vi "quicktest_one_inst.vi"() -> ()   [LabVIEW 2009]
panel:
  out "bucle":i32
  out "Numeric":i32
  out "hex integer string 2":string
  out "IPR value 2":i32
  in  "send continuous":bool
  out "Data out 5":string
  in  "send":bool
  out "hex integer string":string
  out "IPR value":i32
  out "Id in":i32=72
  in  "Read physical":bool
  out "Data to send hex":string
  in  "Register or channel":i32=72
  in  "Device":u16(ring) items=["Attenuation", "Clipping", "Enable channel", "Delay line", "ASIC"]
  in  "Read/#write":bool
  out "data out serial":string
  out "Data to send dec":u32
  in  "Data":i32=72
  out "data out 2":string
  out "error out":errorcluster
  in  "stop":bool
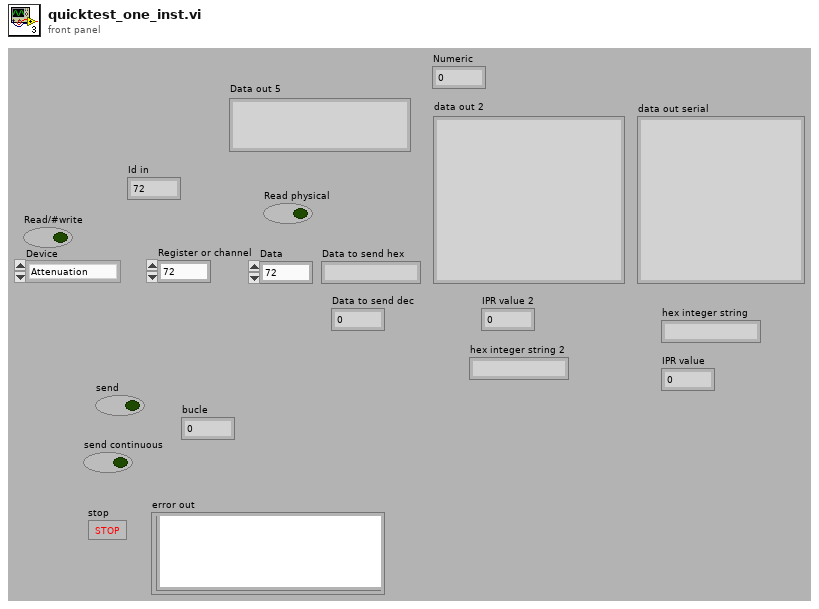
[diagram p1: front panel]
types:
  T1 = enum16{"Standard", "Buffered", "CRLF", "Immediate"}
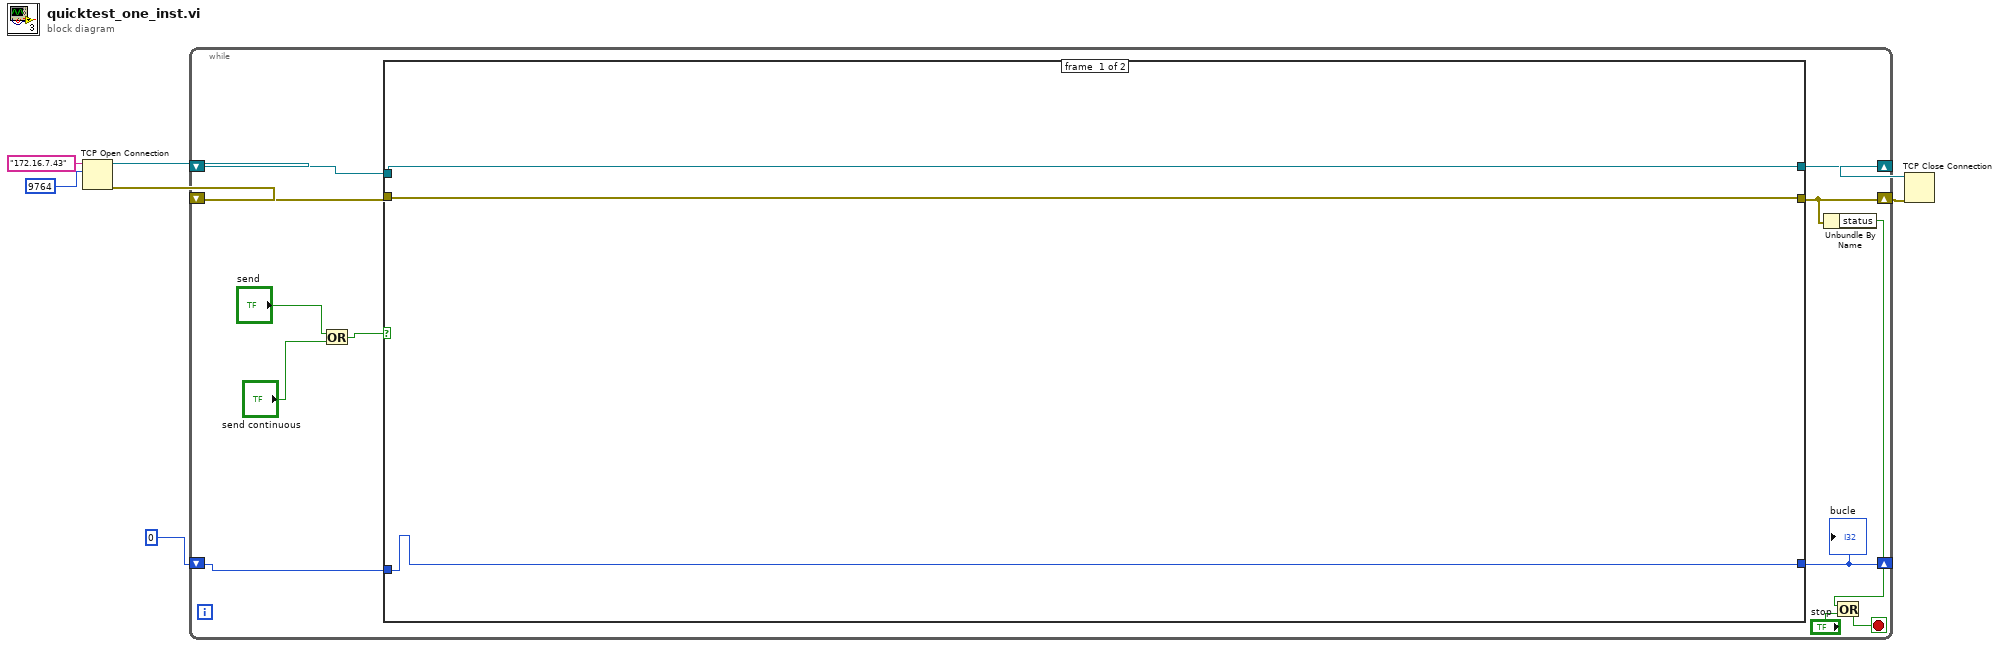
[diagram p0: block diagram]
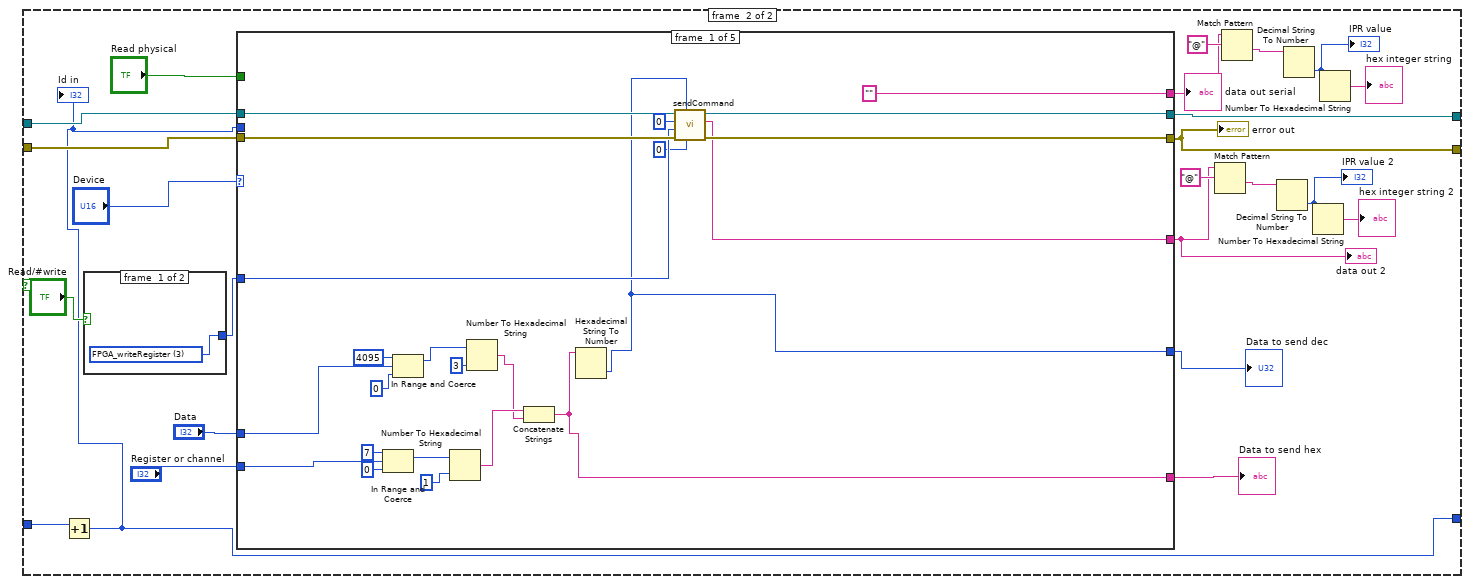
[diagram p2: hidden frame]
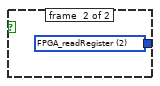
[diagram p3: hidden frame]
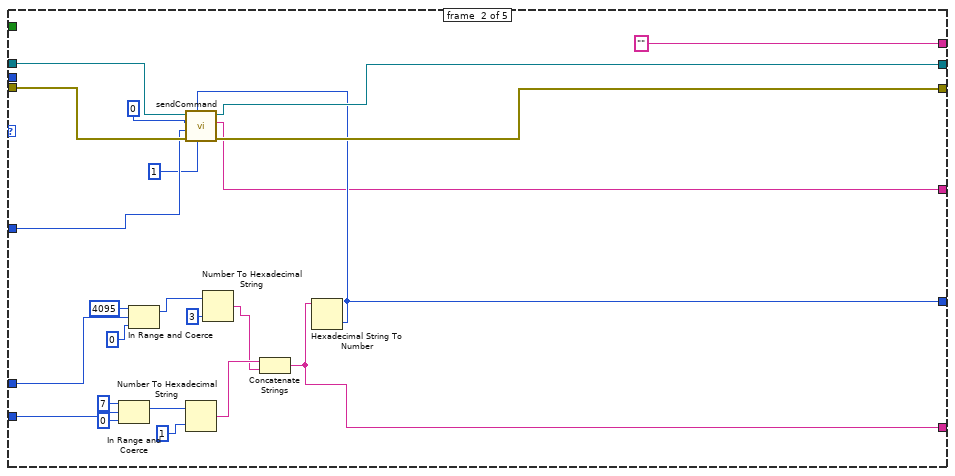
[diagram p4: hidden frame]
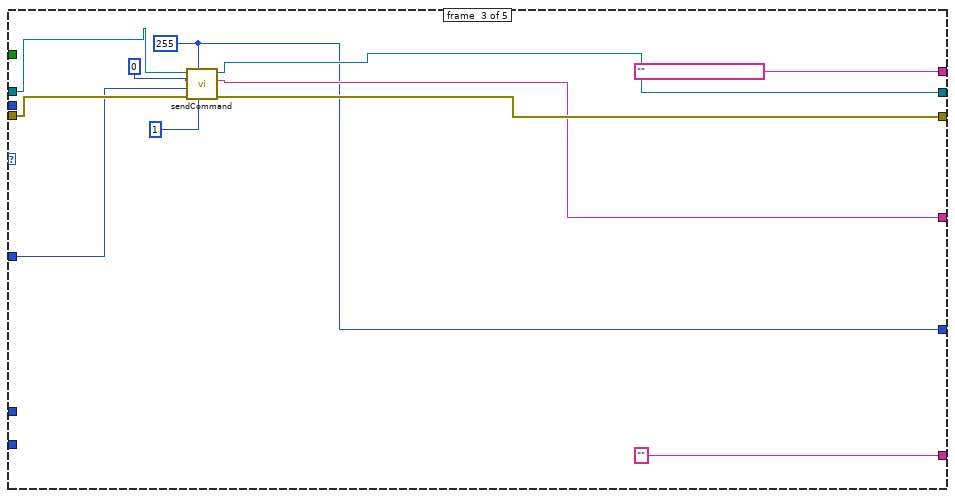
[diagram p5: hidden frame]
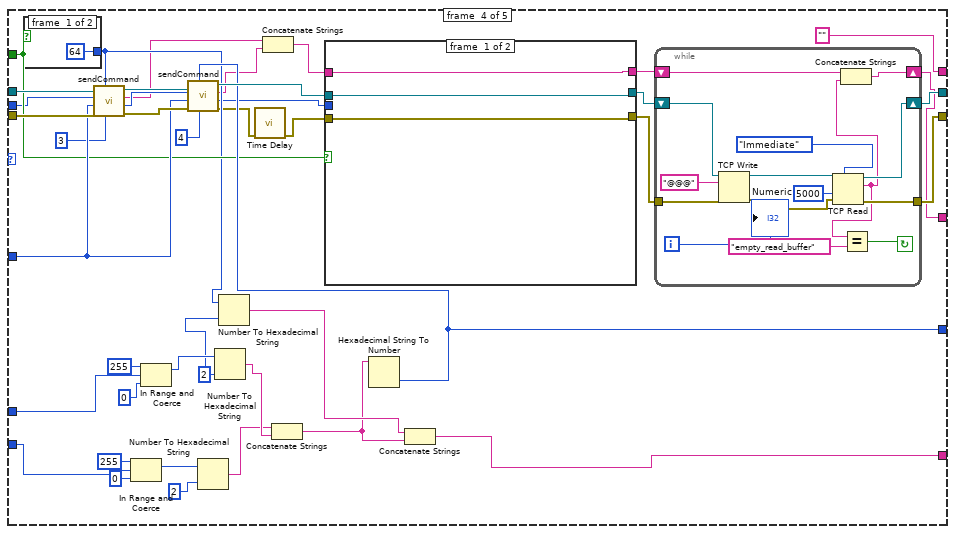
[diagram p6: hidden frame]
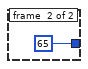
[diagram p7: hidden frame]
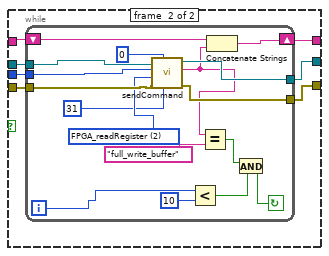
[diagram p8: hidden frame]
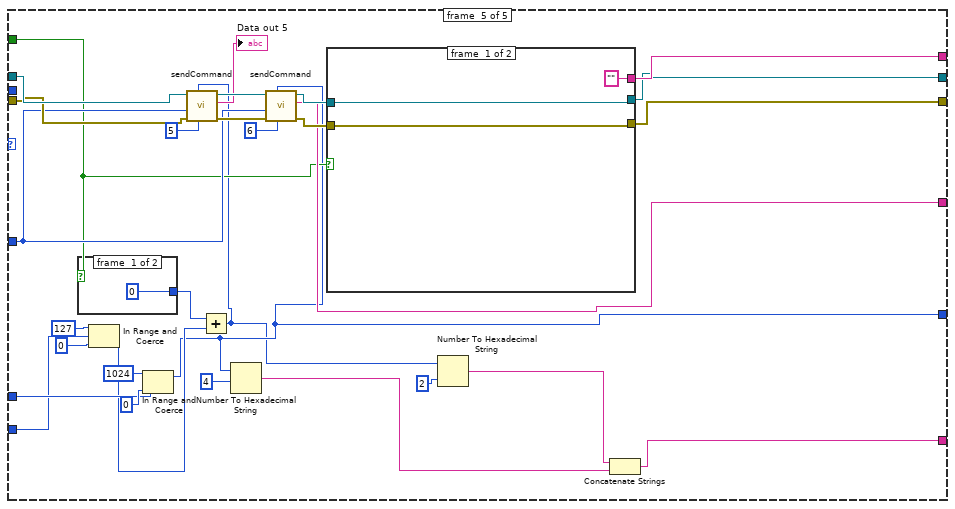
[diagram p9: hidden frame]
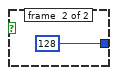
[diagram p10: hidden frame]
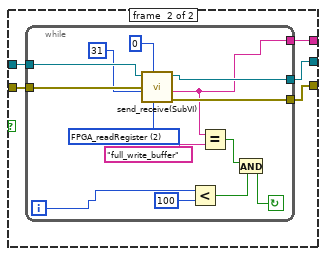
[diagram p11: hidden frame]
diagram:
  n1 = TCP Open Connection(address="172.16.7.43", remote port or service name=u16 9764) -> (connection ID=w3:refnum<k5>, error out=w2:errorcluster)  [unwired: 3 in]
  n2 = while {
    shift-right: [w18] -> w5
    shift-left: w2 -> [w13]
    shift-right: [w19] -> w4
    shift-left: w3 -> [w14]
    shift-right: [w9] -> _
    shift-left: 0 ("lower limit") -> [w8]
    stop <- w17 stop-if-true
    n3 = Or(x="send", y="send continuous") -> (x .or. y?=w10:bool)
    n4 = case shown="True" w10 {
      tunnel: w13 -> [w21 w46]
      tunnel: w14 -> [w22 w45]
      tunnel: [w22 w44] -> w19
      tunnel: [w21 w43] -> w18
      tunnel: [w20 w23] -> w9
      tunnel: w8 -> [w20 w24]
      frame #0 {
      }
      frame #1 {
        n5 = Increment(x=w24) -> (x+1=w23:i32)
        "Id in" <- w23
        n6 = case shown="False" "Read/#write" {
          tunnel: [w47 w48] -> w41
          frame #0 {
            w47 = u16 3 items=["sendCommand"=9, "FPGA_writeRegister"=3, "FPGA_readRegister"=2, "uC_writeRegister"=1, "uC_readRegister"=0] ("Action")
          }
          frame #1 {
            w48 = u16 2 items=["sendCommand"=9, "FPGA_writeRegister"=3, "FPGA_readRegister"=2, "uC_writeRegister"=1, "uC_readRegister"=0] ("Action")
          }
        }
        n7 = case shown="3" "Device" {
          tunnel: [w69 w92 w100 w113 w198] -> w43
          tunnel: w46 -> [w70 w94 w103 w146 w205]
          tunnel: w45 -> [w71 w93 w102 w143 w206]
          tunnel: [w68 w91 w101 w114 w199] -> w44
          tunnel: w41 -> [w56 w88 w97 w142 w204]
          tunnel: "Register or channel" -> [w49 w87 _ w130 w202]
          tunnel: "Data" -> [w50 w82 _ w129 w203]
          tunnel: ["" ("data out") "" ("data out") "" ("data out") "" ("data out") w200] -> w32
          tunnel: [w53 w75 w96 w128 w192] -> w37
          tunnel: [w52 w74 "" w118 w201] -> w36
          tunnel: [w54 w73 w99 w108 w197] -> w25
          tunnel: "Read physical" -> [_ _ _ w127 w196]
          tunnel: w23 -> [_ _ _ w117 _]
          frame #0 {
            n8 = In Range and Coerce(upper limit=7, x=w49, lower limit=0) -> (coerced(x)=w66:i32)  [unwired: 1 out]
            n9 = In Range and Coerce(upper limit=4095, x=w50, lower limit=0) -> (coerced(x)=w62:i32)  [unwired: 1 out]
            n10 = Number To Hexadecimal String(1:i16 1 ("width (-)"), 2:w66) -> (0:w59:string)
            n11 = Number To Hexadecimal String(1:i16 3 ("width (-)"), 2:w62) -> (0:w58:string)
            n12 = Concatenate Strings(w59, w58) -> (w52:string)
            n13 = Hexadecimal String To Number(string=w52) -> (number=w53:u32)  [unwired: 2 in, 1 out]
            n14 = call "sendCommand.vi"("Address"=0, "Data"=w53, "error in"=w70, "Action"=w56, "id_in"=0, "connection ID"=w71) -> ("error out"=w69:errorcluster, "Data out"=w54:string, "connection ID out"=w68:refnum<k5>)  [unwired: 1 in, 2 out]
          }
          frame #1 {
            n15 = In Range and Coerce(upper limit=7, x=w87, lower limit=0) -> (coerced(x)=w86:i32)  [unwired: 1 out]
            n16 = In Range and Coerce(upper limit=4095, x=w82, lower limit=0) -> (coerced(x)=w81:i32)  [unwired: 1 out]
            n17 = Number To Hexadecimal String(1:i16 1 ("width (-)"), 2:w86) -> (0:w78:string)
            n18 = Number To Hexadecimal String(1:i16 3 ("width (-)"), 2:w81) -> (0:w77:string)
            n19 = Concatenate Strings(w78, w77) -> (w74:string)
            n20 = Hexadecimal String To Number(string=w74) -> (number=w75:u32)  [unwired: 2 in, 1 out]
            n21 = call "sendCommand.vi"("Address"=1, "Data"=w75, "error in"=w94, "Action"=w88, "id_in"=0 ("id"), "connection ID"=w93) -> ("error out"=w92:errorcluster, "Data out"=w73:string, "connection ID out"=w91:refnum<k5>)  [unwired: 1 in, 2 out]
          }
          frame #2 {
            w96 = 255 ("Data")
            n22 = call "sendCommand.vi"("Address"=1, "Data"=w96, "error in"=w103, "Action"=w97, "id_in"=0 ("id"), "connection ID"=w102) -> ("error out"=w100:errorcluster, "Data out"=w99:string, "connection ID out"=w101:refnum<k5>)  [unwired: 1 in, 2 out]
          }
          frame #3 {
            w124 = i16 2 ("width (-)")
            n23 = case shown="False" w127 {
              tunnel: [64 ("Address") 65 ("Address")] -> w125
              frame #0 {
              }
              frame #1 {
              }
            }
            n24 = call "sendCommand.vi"("Address"=3, "Data"=w125, "error in"=w146, "Action"=w142, "id_in"=w117, "connection ID"=w143) -> ("error out"=w145:errorcluster, "id_out"=w123:i32, "Data out"=w111:string, "connection ID out"=w144:refnum<k5>)  [unwired: 1 in, 1 out]
            n25 = In Range and Coerce(upper limit=255, x=w130, lower limit=0) -> (coerced(x)=w138:i32)  [unwired: 1 out]
            n26 = In Range and Coerce(upper limit=255, x=w129, lower limit=0) -> (coerced(x)=w134:i32)  [unwired: 1 out]
            n27 = Number To Hexadecimal String(1:i16 2 ("width (-)"), 2:w138) -> (0:w126:string)
            n28 = Number To Hexadecimal String(1:w124, 2:w134) -> (0:w131:string)
            n29 = Number To Hexadecimal String(1:w124, 2:w125) -> (0:w120:string)
            n30 = Concatenate Strings(w126, w131) -> (w119:string)
            n31 = Hexadecimal String To Number(string=w119) -> (number=w128:u32)  [unwired: 2 in, 1 out]
            n32 = call "sendCommand.vi"("Address"=4, "Data"=w128, "error in"=w145, "Action"=w142, "id_in"=w123, "connection ID"=w144) -> ("error out"=w121:errorcluster, "id_out"=w106:i32, "Data out"=w110:string, "connection ID out"=w139:refnum<k5>)  [unwired: 1 in, 1 out]
            n33 = call "Time Delay"("error in (no error)"=w121) -> ("error out"=w122:errorcluster)  [unwired: 10 in]
            n34 = Concatenate Strings(w111, w110) -> (w109:string)
            n35 = case shown="True" w127 {
              tunnel: w139 -> [w165 w173]
              tunnel: w122 -> [w166 w172]
              tunnel: [w166 w169] -> w112
              tunnel: [w165 w170] -> w115
              tunnel: [w164 w171] -> w116
              tunnel: w109 -> [w164 w168]
              tunnel: w106 -> [_ w167]
              frame #0 {
              }
              frame #1 {
                n36 = while {
                  tunnel: w172 -> [w184]
                  tunnel: [w183] -> w169
                  tunnel: [w178] -> w170
                  tunnel: w173 -> [w182]
                  shift-right: [w175] -> w171
                  shift-left: w168 -> [w177]
                  tunnel: w167 -> [w174]
                  i -> [w185]
                  stop <- w186 continue-if-true
                  w181 = u16 2 items=["sendCommand"=9, "FPGA_writeRegister"=3, "FPGA_readRegister"=2, "uC_writeRegister"=1, "uC_readRegister"=0] ("Action 2")
                  n37 = call "sendCommand.vi"("Address"=31, "Data"=0, "error in"=w184, "Action"=w181, "id_in"=w174, "connection ID"=w182) -> ("error out"=w183:errorcluster, "Data out"=w176:string, "connection ID out"=w178:refnum<k5>)  [unwired: 1 in, 2 out]
                  n38 = Less?(x=w185, y=10) -> (x < y?=w188:bool)
                  n39 = Equal?(x=w176, y="full_write_buffer") -> (x = y?=w189:bool)
                  n40 = Concatenate Strings(w177, w176) -> (w175:string)
                  n41 = And(x=w189, y=w188) -> (x .and. y?=w186:bool)
                }
              }
            }
            n42 = Concatenate Strings(w120, w119) -> (w118:string)
            n43 = while {
              tunnel: w112 -> [w156]
              tunnel: [w155] -> w113
              shift-right: [w153] -> w114
              shift-left: w115 -> [w154]
              shift-right: [w151] -> w108
              shift-left: w116 -> [w152]
              i -> [w147]
              stop <- w148 continue-if-true
              n44 = TCP Write(connection ID=w154, data in="@@@", error in (no error)=w156) -> (connection ID out=w160:refnum<k5>, error out=w158:errorcluster)  [unwired: 1 in, 1 out]
              n45 = TCP Read(connection ID=w160, error in (no error)=w158, 7:T1."Immediate" ("mode (standard)"), 9:5000 ("timeout ms (25000)")) -> (connection ID out=w153:refnum<k5>, data out=w150:string, error out=w155:errorcluster)  [unwired: 1 in]
              n46 = Concatenate Strings(w152, w150) -> (w151:string)
              n47 = Equal?(x=w150, y="empty_read_buffer") -> (x = y?=w148:bool)
              "Numeric" <- w147
            }
          }
          frame #4 {
            n48 = case shown="False" w196 {
              tunnel: [0 ("Address") 128 ("Address")] -> w194
              frame #0 {
              }
              frame #1 {
              }
            }
            n49 = In Range and Coerce(upper limit=127, x=w202, lower limit=0) -> (coerced(x)=w193:i32)  [unwired: 1 out]
            n50 = In Range and Coerce(upper limit=1024, x=w203, lower limit=0) -> (coerced(x)=w192:i32)  [unwired: 1 out]
            n51 = Add(x=w194, y=w193) -> (x+y=w191:i32)
            n52 = call "sendCommand.vi"("Address"=5, "Data"=w191, "error in"=w205, "Action"=w204, "connection ID"=w206) -> ("error out"=w220:errorcluster, "Data out"=→"Data out 5":string, "connection ID out"=w219:refnum<k5>)  [unwired: 2 in, 2 out]
            n53 = Number To Hexadecimal String(1:i16 4 ("width (-)"), 2:w192) -> (0:w207:string)
            n54 = call "sendCommand.vi"("Address"=6, "Data"=w192, "error in"=w220, "Action"=w204, "connection ID"=w219) -> ("error out"=w215:errorcluster, "Data out"=w197:string, "connection ID out"=w216:refnum<k5>)  [unwired: 2 in, 2 out]
            n55 = case shown="True" w196 {
              tunnel: w216 -> [w224 w230]
              tunnel: w215 -> [w225 w229]
              tunnel: [w225 w228] -> w198
              tunnel: [w224 w227] -> w199
              tunnel: ["" ("data out") w226] -> w200
              frame #0 {
              }
              frame #1 {
                n56 = while {
                  tunnel: w229 -> [w244]
                  tunnel: [w243] -> w228
                  tunnel: [w242] -> w227
                  tunnel: w230 -> [w241]
                  tunnel: [w231] -> w226
                  i -> [w232]
                  stop <- w233 continue-if-true
                  w239 = u16 2 items=["sendCommand"=9, "FPGA_writeRegister"=3, "FPGA_readRegister"=2, "uC_writeRegister"=1, "uC_readRegister"=0] ("Action 2")
                  n57 = call "send_receive(SubVI).vi"("Action"=w239, "Data"=0, "error in"=w244, "Address"=31, "connection ID"=w241) -> ("error out"=w243:errorcluster, "data out"=w231:string, "connection ID out"=w242:refnum<k5>)  [unwired: 2 in, 2 out]
                  n58 = Less?(x=w232, y=100) -> (x < y?=w235:bool)
                  n59 = Equal?(x=w231, y="full_write_buffer") -> (x = y?=w236:bool)
                  n60 = And(x=w236, y=w235) -> (x .and. y?=w233:bool)
                }
              }
            }
            n61 = Number To Hexadecimal String(1:i16 2 ("width (-)"), 2:w191) -> (0:w208:string)
            n62 = Concatenate Strings(w208, w207) -> (w201:string)
          }
        }
        "error out" <- w43
        "data out serial" <- w32
        "Data to send dec" <- w37
        "Data to send hex" <- w36
        "data out 2" <- w25
        n63 = Match Pattern(string=w25, regular expression="@" ("search string/char (-)")) -> (after substring=w29:string)  [unwired: 1 in, 3 out]
        n64 = Match Pattern(string=w32, regular expression="@" ("search string/char (-)")) -> (after substring=w34:string)  [unwired: 1 in, 3 out]
        n65 = Decimal String To Number(string=w29) -> (number=w27:i32)  [unwired: 2 in, 1 out]
        "IPR value 2" <- w27
        n66 = Decimal String To Number(string=w34) -> (number=w31:i32)  [unwired: 2 in, 1 out]
        "IPR value" <- w31
        n67 = Number To Hexadecimal String(2:w27) -> (0:→"hex integer string 2":string)  [unwired: 1 in]
        n68 = Number To Hexadecimal String(2:w31) -> (0:→"hex integer string":string)  [unwired: 1 in]
      }
    }
    "bucle" <- w9
    n69 = Unbundle By Name(w18) -> ("status"=w16:bool)
    n70 = Or(x=w16, y="stop") -> (x .or. y?=w17:bool)
  }
  n71 = TCP Close Connection(connection ID=w4, error in (no error)=w5) -> ()  [unwired: 1 in, 2 out]
